vi "Image to Info.vi"(8 "error in (no error)":errorcluster, 11 "Front Panel":T2) -> (0 "error out":errorcluster, 3 "Image Info":T1)   [LabVIEW 2021, in "NI Measurement Plug-In SDK.lvlib" / "VI Info.lvlib"]
uses:
  VI Info.lvlib
  <vilib>/picture/picture.llb/imagedata.ctl
  Image Info.ctl
  <vilib>/wsapi/NI_WebServices.lvlib
  <vilib>/JDP Science/JDP Science Common Utilities/Base64/Base64 Support.lvlib
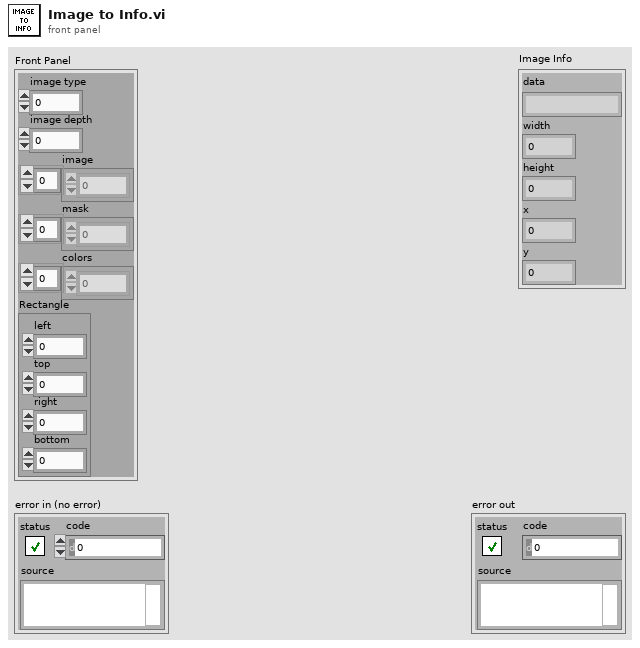
[diagram p1: front panel]
types:
  T1 = typedef "NI Measurement Plug-In SDK.lvlib/VI Info.lvlib/Image Info.ctl" = cluster{"data":string, "width":i16, "height":i16, "x":i16, "y":i16}
  T2 = typedef "imagedata.ctl" = cluster{"image type":i32, "image depth":i32, "image":u8[], "mask":u8[], "colors":u32[], "Rectangle":cluster{"left":i16, "top":i16, "right":i16, "bottom":i16}}
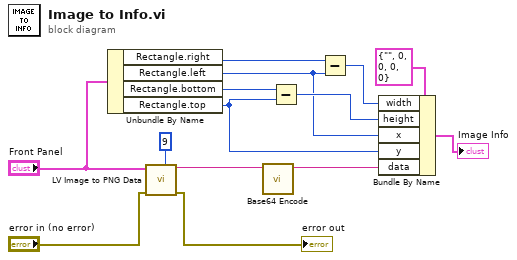
[diagram p0: block diagram]
diagram:
  n1 = Unbundle By Name("Front Panel") -> ("Rectangle.right"=w7:i16, "Rectangle.left"=w3:i16, "Rectangle.bottom"=w8:i16, "Rectangle.top"=w2:i16)
  n2 = call <vilib>:"LV Image to PNG Data.vi"("compression (none)"=9, "error in (no error)"="error in (no error)", "image data"="Front Panel") -> ("error out"=→"error out":errorcluster, "png data"=w6:string)  [unwired: 7 in]
  n3 = call <vilib>:"Base64 Encode.vi"("String to Encode"=w6) -> ("Base64 Encoded"=w1:string)  [unwired: 10 in]
  n4 = Subtract(x=w8, y=w2) -> (x-y=w4:i16)
  n5 = Subtract(x=w7, y=w3) -> (x-y=w5:i16)
  n6 = Bundle By Name(cluster=T1 {"data"="", "width"=0, "height"=0, "x"=0, "y"=0} ("Image Info"), "width"=w5, "height"=w4, "x"=w3, "y"=w2, "data"=w1) -> (→"Image Info":T1)
